vi "Fill To.vi"(5 "Col":i32, 6 "Attributes":T1, 7 "Row":i32, 8 "error in (no error)":errorcluster, 10 "Char":string, 11 "TermBuffer in":refnum<class "TermBuffer.lvclass">) -> (0 "error out":errorcluster, 3 "TermBuffer out":refnum<class "TermBuffer.lvclass">)   [LabVIEW 2020, in "Terminal.lvlib" / "TermBuffer.lvclass"]
uses:
  TermBuffer.lvclass
  TermBuffer.lvclass/TermBuffer.ctl
  TermLine/TermLine.lvclass
  Text Attributes.ctl
  Terminal.lvlib
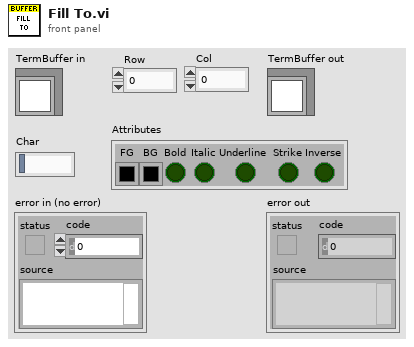
[diagram p1: front panel]
types:
  T1 = typedef "Terminal.lvlib/Text Attributes.ctl" = cluster{"FG":u32, "BG":u32, "Bold":bool, "Italic":bool, "Underline":bool, "Strike":bool, "Inverse":bool}
  T2 = typedef "Terminal.lvlib/TermBuffer.lvclass/Ref Data.ctl" = cluster{"Lines":refnum<class "TermLine.lvclass">[], "Rows":i32, "Cols":i32}
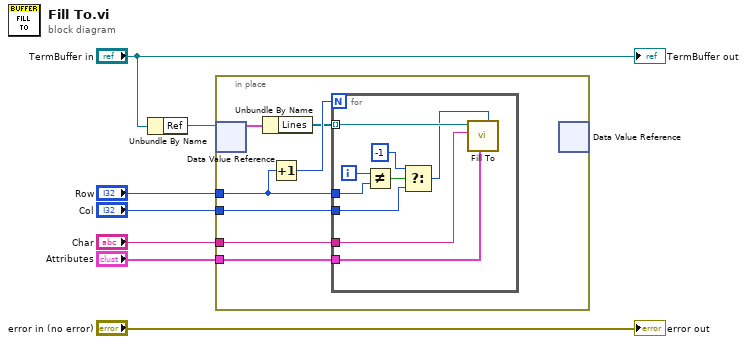
[diagram p0: block diagram]
diagram:
  n1 = Unbundle By Name("TermBuffer in") -> ("Ref"=w6:refnum<data-value>)
  n2 = in-place {
    in-place-border: "Row" -> [w11]
    in-place-border: "Col" -> [w10]
    in-place-border: "Char" -> [w9]
    in-place-border: "Attributes" -> [w8]
    n3 = in-place-dvr #1(w6) -> (w14:T2)  [unwired: 1 out]
    n4 = Unbundle By Name(w14) -> ("Lines"=w12:refnum<class "TermLine.lvclass">[])
    n5 = Increment(x=w11) -> (x+1=w13:i32)
    n6 = for {
      N: w13 -> [_]
      tunnel: w12 -> [w21] mode=indexing
      tunnel: w11 -> [w23]
      tunnel: w10 -> [w19]
      tunnel: w9 -> [w16]
      tunnel: w8 -> [w15]
      i -> [w22]
      n7 = Not Equal?(x=w22, y=w23) -> (x != y?=w20:bool)
      n8 = Select(t=-1, s=w20, f=w19) -> (s? t:f=w17:i32)
      n9 = call "Fill To.vi"("Col"=w17, "Attributes"=w15, "Char"=w16, "TermLine in"=w21) -> ()  [unwired: 6 in, 2 out]
    }
    n10 = in-place-dvr #1() -> ()  [unwired: 1 in, 2 out]
  }
  "error out" <- "error in (no error)"
  "TermBuffer out" <- "TermBuffer in"
